vi "Gas Thermal Check Basic Tolerance.vi"(0 "Inlet Temperature (F) - Target":dbl, 1 "Target RTDout-RTDin":dbl, 2 "Temperature +- Tolerance (F)":dbl, 5 "RTD Out (Deg F)":dbl, 9 "RTD In (Deg F)":dbl, 11 "error in (no error)":errorcluster) -> (4 "RTDin Stable":bool, 6 "RTDout Stable":bool, 10 "RTDout-RTDin Stable":bool, 15 "error out":errorcluster)   [LabVIEW 2019]
panel:
  out "RTDout-RTDin":dbl
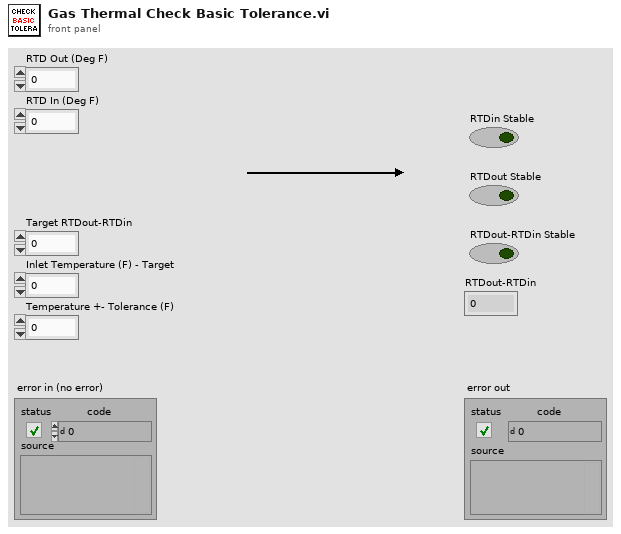
[diagram p1: front panel]
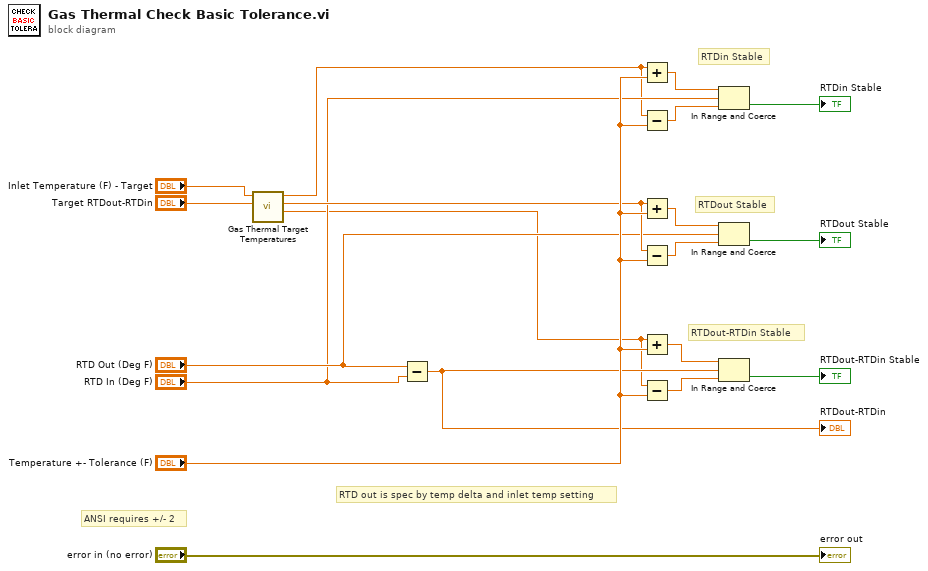
[diagram p0: block diagram]
diagram:
  # "RTD out is spec by temp delta and inlet temp setting"
  # "ANSI requires +/- 2"
  # "RTDout-RTDin Stable"
  # "RTDout Stable"
  # "RTDin Stable"
  n1 = call "Gas Thermal Target Temperatures.vi"("Target RTDout-RTDin in"="Target RTDout-RTDin", "Inlet Temperature (F) - Target in"="Inlet Temperature (F) - Target") -> ("Target RTDout-RTDin out"=w4:dbl, "Target RTDout"=w11:dbl, "Target Inlet Temperature (F)"=w7:dbl)  [unwired: 6 in, 1 out]
  n2 = Subtract(x="RTD Out (Deg F)", y="RTD In (Deg F)") -> (x-y=w8:dbl)
  "RTDout-RTDin" <- w8
  n3 = Add(x=w7, y="Temperature +- Tolerance (F)") -> (x+y=w5:dbl)
  n4 = Subtract(x=w7, y="Temperature +- Tolerance (F)") -> (x-y=w6:dbl)
  n5 = Add(x=w11, y="Temperature +- Tolerance (F)") -> (x+y=w12:dbl)
  n6 = Subtract(x=w11, y="Temperature +- Tolerance (F)") -> (x-y=w13:dbl)
  n7 = Add(x=w4, y="Temperature +- Tolerance (F)") -> (x+y=w15:dbl)
  n8 = Subtract(x=w4, y="Temperature +- Tolerance (F)") -> (x-y=w14:dbl)
  n9 = In Range and Coerce(upper limit=w5, x="RTD In (Deg F)", lower limit=w6) -> (In Range?=→"RTDin Stable":bool)  [unwired: 1 out]
  n10 = In Range and Coerce(upper limit=w12, x="RTD Out (Deg F)", lower limit=w13) -> (In Range?=→"RTDout Stable":bool)  [unwired: 1 out]
  n11 = In Range and Coerce(upper limit=w15, x=w8, lower limit=w14) -> (In Range?=→"RTDout-RTDin Stable":bool)  [unwired: 1 out]
  "error out" <- "error in (no error)"
